vi "oa_Analog Tacho Hysteresis (No State).vi"(0 "input signal":dbl[](array[numeric]), 1 "reset? (T)":bool=TRUE, 5 "threshold (auto)":dbl=inf format="%.2f", 7 "slope (Rising)":u16(ring) items=["Rising", "Falling"], 9 "hysteresis(0)":dbl format="%.2f", 11 "error in (no error)":errorcluster, 12 "last value in":dbl) -> (4 "output signal":dbl[](array[numeric]), 14 "last value out":dbl, 15 "error out":errorcluster)   [LabVIEW 2012, in "Measurement Channels.lvlib" / "Tachometer.lvclass"]
doc: "This VI works like a hysteresis comparater. It can transform the input tachometer signal into a standard square waveform, ignoring small pulsed caused by harmonics or noise. By setting the hystersis value properly, it can make the speed tracking more accurately."
uses:
  Tachometer.lvclass
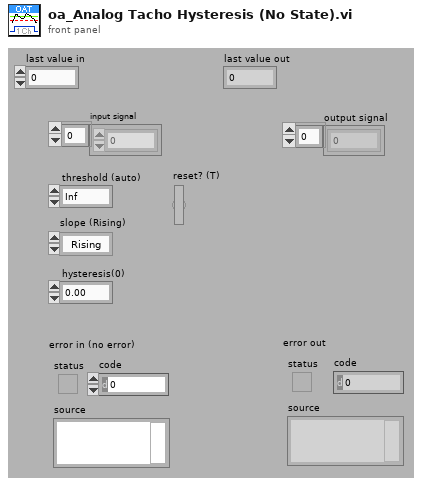
[diagram p1: front panel]
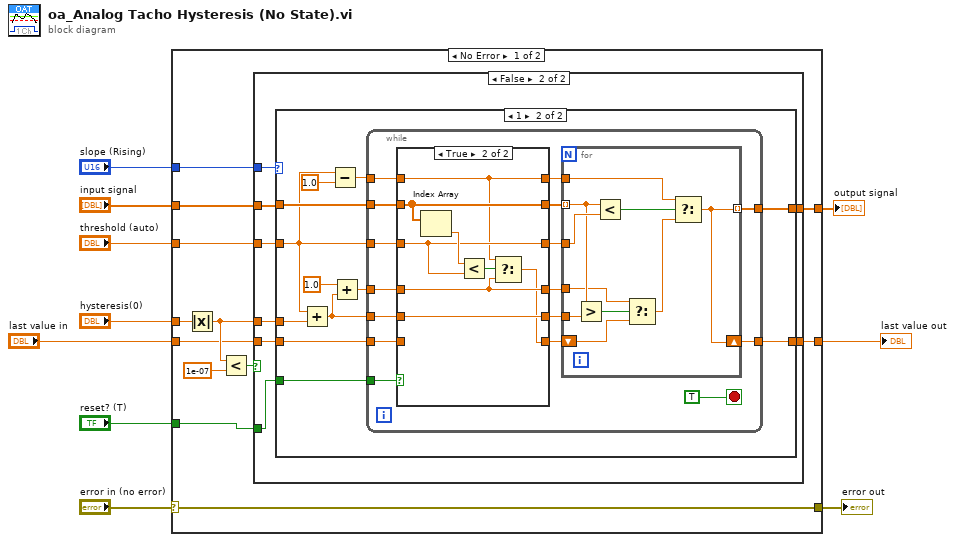
[diagram p0: block diagram]
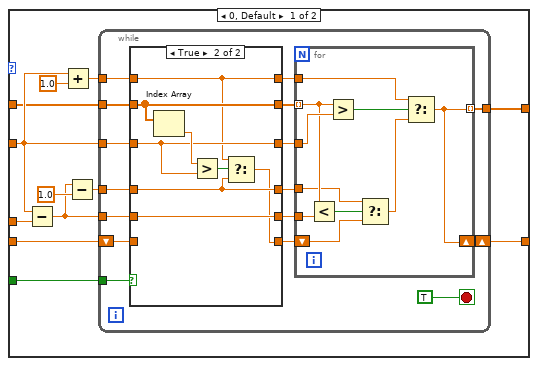
[diagram p3: hidden frame]
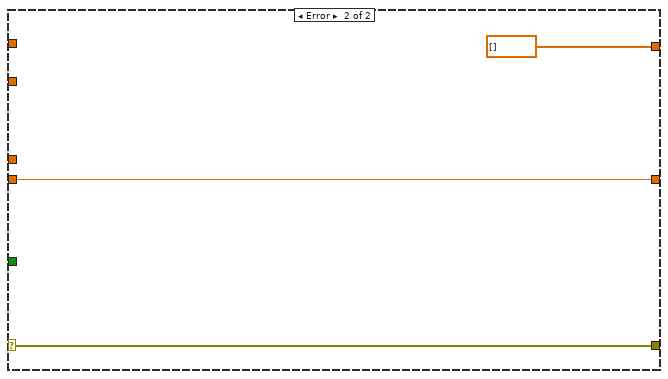
[diagram p6: hidden frame]
diagram:
  n1 = case shown="No Error" "error in (no error)" {
    selector: "error in (no error)" -> [w18 w139]
    tunnel: "reset? (T)" -> [w13 _]
    tunnel: "hysteresis(0)" -> [w14 _]
    tunnel: "threshold (auto)" -> [w21 _]
    tunnel: "slope (Rising)" -> [w20 _]
    tunnel: [w19 dbl[] [] ("signal")] -> w3
    tunnel: [w18 w139] -> w5
    tunnel: "input signal" -> [w17 _]
    tunnel: "last value in" -> [w12 w137]
    tunnel: [w11 w137] -> w1
    frame No Error {
      n2 = Absolute Value(x=w14) -> (abs(x)=w15:dbl)
      n3 = Less?(x=w15, y=1e-07) -> (x < y?=w22:bool)
      n4 = case shown="False" w22 {
        tunnel: w17 -> [w24 w29]
        tunnel: [w24 w28] -> w19
        tunnel: w15 -> [_ w27]
        tunnel: w20 -> [_ w32]
        tunnel: w21 -> [_ w31]
        tunnel: w13 -> [_ w30]
        tunnel: w12 -> [w23 w26]
        tunnel: [w23 w25] -> w11
        frame True {
        }
        frame False {
          n5 = case shown="1" w32 {
            tunnel: w29 -> [w37 w96]
            tunnel: w31 -> [w39 w92]
            tunnel: w27 -> [w43 w93]
            tunnel: w30 -> [w36 w87]
            tunnel: [w35 w88] -> w28
            tunnel: w26 -> [w34 w86]
            tunnel: [w33 w85] -> w25
            frame 0, Default {
              n6 = Subtract(x=w39, y=w43) -> (x-y=w41:dbl)
              n7 = Add(x=w39, y=1.0) -> (x+y=w38:dbl)
              n8 = Subtract(x=w41, y=1.0) -> (x-y=w42:dbl)
              n9 = while {
                tunnel: w39 -> [w52]
                tunnel: w37 -> [w50]
                shift-right: [w59] -> w33
                shift-left: w34 -> [w46]
                tunnel: [w58] -> w35
                tunnel: w42 -> [w54]
                tunnel: w41 -> [w56]
                tunnel: w38 -> [w48]
                tunnel: w36 -> [w57]
                stop <- TRUE stop-if-true
                n10 = case shown="True" w57 {
                  tunnel: w56 -> [w65 w74]
                  tunnel: [w65 w74] -> w55
                  tunnel: w54 -> [w64 w68]
                  tunnel: [w64 w68] -> w53
                  tunnel: w52 -> [w63 w71]
                  tunnel: [w63 w71] -> w51
                  tunnel: w50 -> [w62 w73]
                  tunnel: [w62 w73] -> w49
                  tunnel: w48 -> [w61 w69]
                  tunnel: [w61 w69] -> w47
                  tunnel: w46 -> [w66 _]
                  tunnel: [w66 w67] -> w45
                  frame False {
                  }
                  frame True {
                    n11 = Index Array(array=w73) -> (element=w72:dbl)  [unwired: 1 in]
                    n12 = Greater?(x=w72, y=w71) -> (0:w70:bool)
                    n13 = Select(t=w69, s=w70, f=w68) -> (s? t:f=w67:dbl)
                  }
                }
                n14 = for {
                  tunnel: w49 -> [w82] mode=indexing
                  tunnel: w51 -> [w84]
                  shift-right: [w75] -> w59
                  shift-left: w45 -> [w76]
                  tunnel: w55 -> [w80]
                  tunnel: w47 -> [w79]
                  tunnel: w53 -> [w77]
                  tunnel: [w75] -> w58 mode=indexing
                  n15 = Less?(x=w82, y=w80) -> (x < y?=w81:bool)
                  n16 = Greater?(x=w82, y=w84) -> (0:w83:bool)
                  n17 = Select(t=w77, s=w81, f=w76) -> (s? t:f=w78:dbl)
                  n18 = Select(t=w79, s=w83, f=w78) -> (s? t:f=w75:dbl)
                }
              }
            }
            frame 1 {
              n19 = Add(x=w92, y=w93) -> (x+y=w89:dbl)
              n20 = Subtract(x=w92, y=1.0) -> (x-y=w95:dbl)
              n21 = Add(x=1.0, y=w89) -> (x+y=w90:dbl)
              n22 = while {
                tunnel: w92 -> [w104]
                tunnel: w96 -> [w102]
                tunnel: [w110] -> w88
                tunnel: w90 -> [w106]
                tunnel: w89 -> [w108]
                tunnel: w95 -> [w100]
                tunnel: w87 -> [w109]
                tunnel: w86 -> [w98]
                tunnel: [w111] -> w85
                stop <- TRUE stop-if-true
                n23 = case shown="True" w109 {
                  tunnel: w108 -> [w117 w126]
                  tunnel: [w117 w126] -> w107
                  tunnel: w106 -> [w116 w120]
                  tunnel: [w116 w120] -> w105
                  tunnel: w104 -> [w115 w123]
                  tunnel: [w115 w123] -> w103
                  tunnel: w102 -> [w114 w125]
                  tunnel: [w114 w125] -> w101
                  tunnel: w100 -> [w113 w121]
                  tunnel: [w113 w121] -> w99
                  tunnel: w98 -> [w118 _]
                  tunnel: [w118 w119] -> w97
                  frame False {
                  }
                  frame True {
                    n24 = Index Array(array=w125) -> (element=w124:dbl)  [unwired: 1 in]
                    n25 = Less?(x=w124, y=w123) -> (x < y?=w122:bool)
                    n26 = Select(t=w121, s=w122, f=w120) -> (s? t:f=w119:dbl)
                  }
                }
                n27 = for {
                  tunnel: w101 -> [w134] mode=indexing
                  tunnel: w103 -> [w136]
                  shift-right: [w127] -> w111
                  shift-left: w97 -> [w128]
                  tunnel: w107 -> [w132]
                  tunnel: w99 -> [w131]
                  tunnel: w105 -> [w129]
                  tunnel: [w127] -> w110 mode=indexing
                  n28 = Greater?(x=w134, y=w132) -> (0:w133:bool)
                  n29 = Less?(x=w134, y=w136) -> (x < y?=w135:bool)
                  n30 = Select(t=w129, s=w133, f=w128) -> (s? t:f=w130:dbl)
                  n31 = Select(t=w131, s=w135, f=w130) -> (s? t:f=w127:dbl)
                }
              }
            }
          }
        }
      }
    }
    frame Error {
    }
  }
  "error out" <- w5
  "output signal" <- w3
  "last value out" <- w1
